vi "NanotecSMCPD.close.vi"(0 "i ref in":refnum<vi>, 5 "error in (no error)":errorcluster) -> (14 "i ref out":refnum<vi>, 19 "error out":errorcluster)   [LabVIEW 2014, in "NanotecSMCPD.lvlib"]
doc: "Closes the VISA interface to the controller."
uses:
  NanotecSMCPD.lvlib
  CS_Core/CSSystem/CoreDefs/CoreDefs.error_type.ctl
  CS_Core/CSSystem/CoreDefs/CoreDefs.error_severity.ctl
  CS_Core/CSApplicationBaseClasses/MotorBase/MotorBase.directionType.ctl
  CS_Core/CSApplicationBaseClasses/MotorBase/MotorBase.serviceType.ctl
  CS_Core/CSApplicationBaseClasses/DeviceBase/DeviceBase.deviceState.ctl
  CS_Core/CSApplicationBaseClasses/MotorBase/MotorBase.lvlib
  CS_Core/CSSystem/CoreLib/CoreLib.lvlib
  CS_Core/CSApplicationBaseClasses/DeviceBase/DeviceBase.lvlib
  instr.lib/NanotecSMCPD/NanotecSMCPDDriver.lvlib
  CSlibraries/UtilityLib/UtilityLib.lvlib
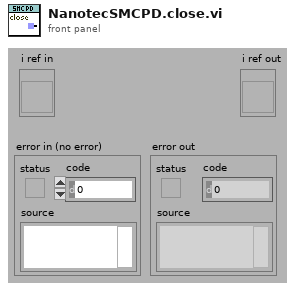
[diagram p1: front panel]
types:
  T1 = typedef "CoreDefs.error_severity.ctl" = enum16{"undefined", "information", "warning", "error", "fatal"}
  T2 = typedef "CoreDefs.error_type.ctl" = enum16{"no error", "can't load process", "can't unload process", "process does not exist", "can't install process", "can't remove process", "unknown function", "time out", "can't execute function", "duplicate queue name", "super not found", "caller queue invalid", "can't ping process", "unknown error", "VISA Error", "VISA timeout", "GPIB timeout", "GPIB error", "communication error", "data type mismatch", "can't read data from OPC server", "can't write data to OPC server", "OET error", "function not implemented", "process already exists", "invalid Shared Variable name", "error writing Shared Variable", "error reading Shared Variable", "invalid client name", "corrupt database", "unknown class", "call not authorized", "parameter out of range", "OET timeout: can't get data to modify", "invalid queue name", "requested operation incompatible with current state", "event undefined", "event disabled", "state undefined", "caller is not a friend", "EventBuilder: bad eventID", "EventBuilder: no DAQ devices", "a thread must not stop itself", "UNUSED ELEMENT4", "DiscArchiver: eventData incomplete", "DiscArchiver: eventData does not belong to run", "DiscArchiver: can't open file", "DiscArchiver: can't write to file", "DiscArchiver: available disc space low", "can't acquire semaphore", "error reading data from database", "notifier object is not existing", "can't register process", "can't unregister process", "illegal event type", "object disabled", "object already exists", "can't change state", "Instrument not found", "no connection to remote node", "invalid reference", "N/A", "UNUSED ELEMENT 1", "element not found", "illegal TCP/IP connection detected", "object does not exist", "invalid access ID", "unknown CS system", "invalid privilige", "unsupported data type", "unsupported server type", "IO server already exists", "Shared Variable already exists"}
  T3 = typedef "MotorBase.lvlib/MotorBase.serviceType.ctl" = enum16{"onOff", "startVelocity", "stopVelocity", "acceleration", "rangeMin", "rangeMax", "status", "position"}
  T4 = typedef "MotorBase.lvlib/MotorBase.directionType.ctl" = enum16{"unknown", "update actual value", "update nominal value", "update both"}
  T5 = typedef "DeviceBase.lvlib/DeviceBase.deviceState.ctl" = i16
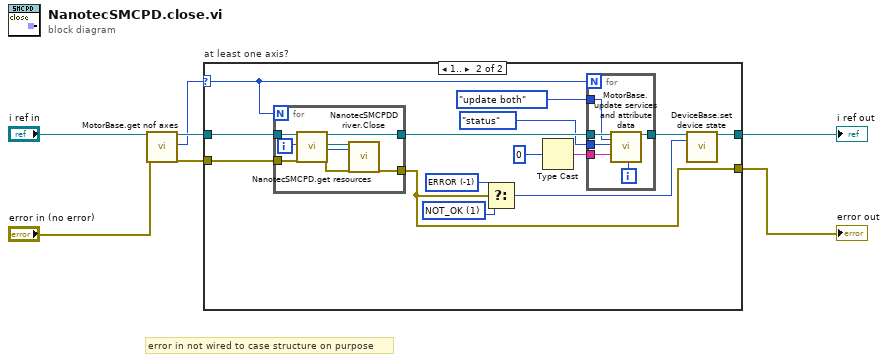
[diagram p0: block diagram]
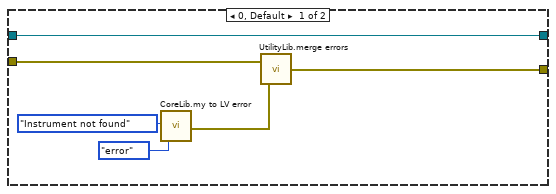
[diagram p2: hidden frame]
diagram:
  # "error in not wired to case structure on purpose"
  n1 = call "MotorBase.get nof axes.vi"("i ref in"="i ref in", "error in (no error)"="error in (no error)") -> ("i ref out"=w3:refnum<vi>, "nOfAxis"=w1:i32, "error out"=w2:errorcluster)  [unwired: 15 in]
  n2 = case "at least one axis?" shown="1.." w1 {
    selector: w1 -> [_ w14]
    tunnel: w3 -> [w13 w26]
    tunnel: w2 -> [w8 w27]
    tunnel: [w13 w25] -> w6
    tunnel: [w9 w15] -> w5
    frame 0, Default {
      n3 = call "CoreLib.my to LV error.vi"("ErrorTypes"=CoreDefs.error_type."Instrument not found", "severityLevel"=CoreDefs.error_severity."error") -> ("myErrorCluster"=w10:errorcluster)  [unwired: 16 in, 1 out]
      n4 = call "UtilityLib.merge errors.vi"("error2 (no error)"=w10, "error1 (no error)"=w8) -> ("error out"=w9:errorcluster)
    }
    frame 1.. {
      w17 = T5 1 items=["ERROR"=-1, "OK"=0, "NOT_OK"=1] ("deviceState")
      w18 = T5 -1 items=["ERROR"=-1, "OK"=0, "NOT_OK"=1] ("deviceState")
      n5 = for {
        N: w14 -> [_]
        tunnel: w27 -> [w35]
        tunnel: w26 -> [w34]
        tunnel: [w32] -> w24
        tunnel: [w31] -> w15
        i -> [w28]
        n6 = call "NanotecSMCPD.get resources.vi"("i ref in"=w34, "axisNumber"=w28, "error in (no error)"=w35) -> ("i ref out"=w32:refnum<vi>, "VISA resource"=w30:refnum<visa-resource-name>, "address"=w29:i32, "error out"=w33:errorcluster)  [unwired: 13 in]
        n7 = call "NanotecSMCPDDriver.Close.vi"("VISA resource name"=w30, "contollerID"=w29, "error in (no error)"=w33) -> ("error out"=w31:errorcluster)  [unwired: 16 in]
      }
      n8 = Select(t=w18, s=w15, f=w17) -> (s? t:f=w16:T5)
      n9 = Type Cast(x=0) -> (*(type *) &x=w19:string)  [unwired: 1 in]
      n10 = for {
        N: w14 -> [_]
        tunnel: w24 -> [w41]
        tunnel: [w40] -> w23
        tunnel: MotorBase.directionType."update both" ("direction") -> [w39]
        tunnel: MotorBase.serviceType."status" ("service") -> [w38]
        tunnel: w19 -> [w36]
        i -> [w37]
        n11 = call "MotorBase.update services and attribute data.vi"("i ref in"=w41, "direction"=w39, "service"=w38, "value"=w36, "axisNumber"=w37) -> ("i ref out"=w40:refnum<vi>)  [unwired: 12 in, 2 out]
      }
      n12 = call "DeviceBase.set device state.vi"("i ref in"=w23, "deviceState"=w16) -> ("i ref out"=w25:refnum<vi>)  [unwired: 15 in, 2 out]
    }
  }
  "error out" <- w5
  "i ref out" <- w6
